vi "DoCreateError.vi"(6 "AdditionalText":string, 7 "Data":variant, 8 "ErrorIn":errorcluster caption="Error In", 9 "Text":string, 10 "ErrorCode":i32, 11 "ObjectIn":refnum<class "ErrorCreationMGI.lvclass"> caption="Object In") -> (0 "ErrorOut":errorcluster caption="Error Out", 3 "ObjectOut":refnum<class "ErrorCreationMGI.lvclass"> caption="Object Out")   [LabVIEW 2018, in "ErrorCreationMGI.lvclass"]
uses:
  <userlib>/_express/CustomErrorCreator/ErrorCreationTypes/ErrorCreationMGI/ErrorCreationMGI.lvclass
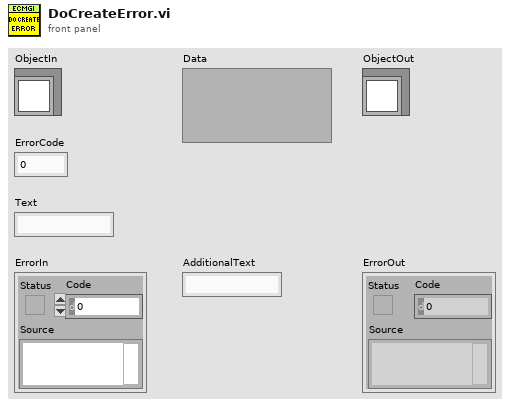
[diagram p1: front panel]
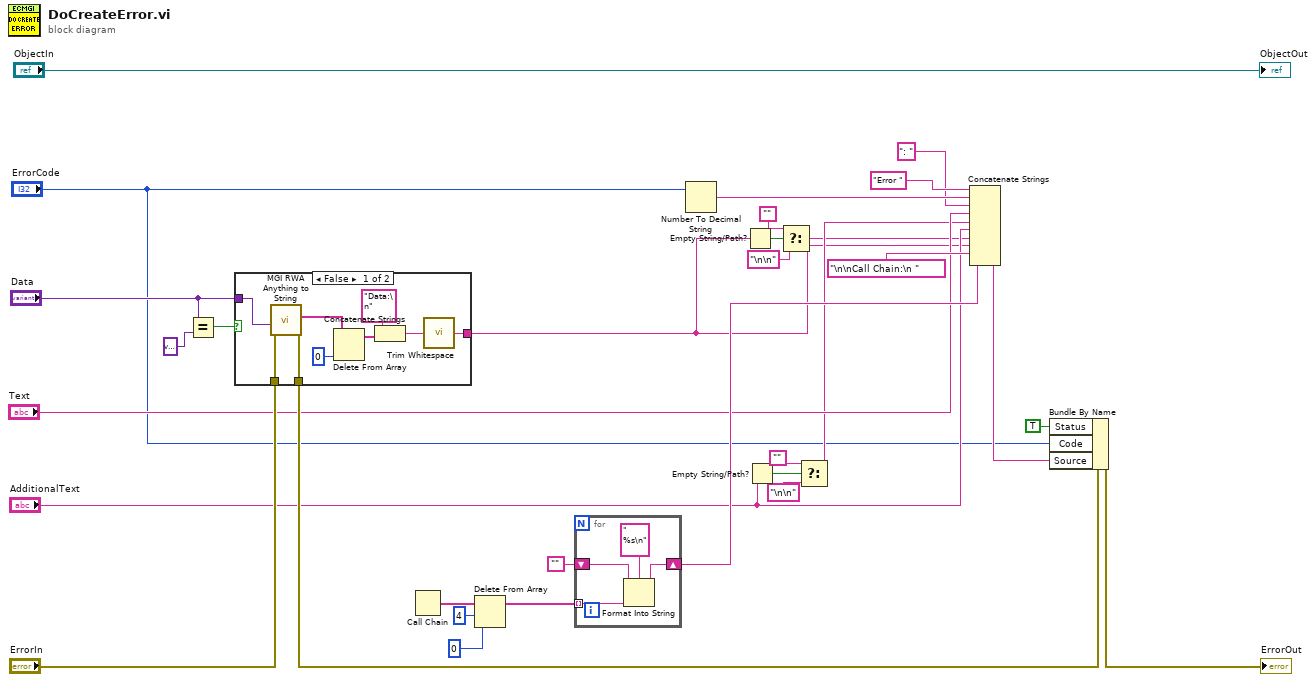
[diagram p0: block diagram]
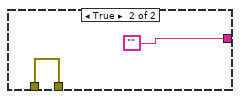
[diagram p2: hidden frame]
diagram:
  n1 = Equal?(x="Data", y=variant) -> (x = y?=w25:bool)
  n2 = case shown="False" w25 {
    tunnel: [w32 ""] -> w4
    tunnel: "Data" -> [w36 _]
    tunnel: "ErrorIn" -> [w34 w41]
    tunnel: [w33 w41] -> w24
    frame False {
      n3 = call <userlib>:"MGI RWA Anything to String.vi"("Error In"=w34, "Anything"=w36) -> ("Error Out"=w33:errorcluster, "Strings[]"=w39:string[])  [unwired: 6 in, 2 out]
      n4 = Delete From Array(array=w39, index=0) -> (array with subset deleted=w40:string[])  [unwired: 1 in, 1 out]
      n5 = Concatenate Strings("Data:\n" ("string"), w40) -> (w37:string)
      n6 = call <vilib>:"Trim Whitespace.vi"("string"=w37) -> ("trimmed string"=w32:string)  [unwired: 1 in]
    }
    frame True {
    }
  }
  n7 = Call Chain() -> (call chain=w22:string[])
  n8 = Delete From Array(array=w22, length=4, index=0 ("length")) -> (array with subset deleted=w21:string[])  [unwired: 1 out]
  n9 = for {
    tunnel: w21 -> [w46] mode=indexing
    shift-right: [w44] -> w14
    shift-left: "" -> [w45]
    n10 = Format Into String(format string="  %s\n", initial string=w45, w46) -> (resulting string=w44:string)  [unwired: 1 in, 1 out]
  }
  n11 = Number To Decimal String(number="ErrorCode") -> (decimal integer string=w17:string)  [unwired: 1 in]
  n12 = Empty String/Path?(string/path=w4) -> (empty?=w8:bool)
  n13 = Empty String/Path?(string/path="AdditionalText") -> (empty?=w11:bool)
  n14 = Select(t="", s=w8, f="\n\n") -> (s? t:f=w5:string)
  n15 = Select(t="", s=w11, f="\n\n") -> (s? t:f=w7:string)
  n16 = Concatenate Strings("Error " ("format string"), w17, ": " ("format string"), "Text", w7, "AdditionalText", w5, w4, "\n\nCall Chain:\n " ("format string"), w14) -> (w13:string)
  n17 = Bundle By Name(cluster=w24, "Status"=TRUE ("status"), "Code"="ErrorCode", "Source"=w13) -> (→"ErrorOut":errorcluster)
  "ObjectOut" <- "ObjectIn"
